vi "Validate Name Is Unique.vi"(8 "error in (no error)":errorcluster, 10 "Name in":string, 11 "Parent Ref in":T1=18446744073709551615 format="%.0x") -> (0 "error out":errorcluster, 1 "Unique?":bool, 2 "Name out":string, 3 "Parent Ref out":T1=18446744073709551615 format="%.0x")   [LabVIEW 2018, in "Instrument Addon Scripting API.lvlib"]
uses:
  Instrument Addon Scripting API.lvlib
  <vilib>/NI Veristand/Custom Device API/Custom Device Item Ref.ctl
  <vilib>/NI Veristand/Custom Device Tools/Custom Device Utility Library/Custom Device Utility Library.lvlib
  <vilib>/NI Veristand/Custom Device API/Custom Device API.lvlib
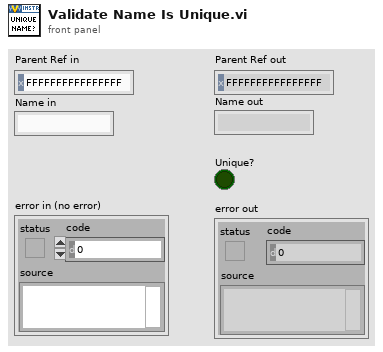
[diagram p1: front panel]
types:
  T1 = typedef "Custom Device API.lvlib/Custom Device Item Ref.ctl" = u64
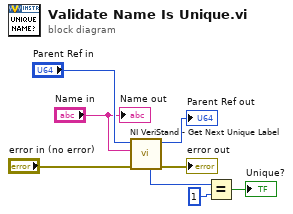
[diagram p0: block diagram]
diagram:
  n1 = call <vilib>:"NI VeriStand - Get Next Unique Label.vi"("error in (no error)"="error in (no error)", "Label"="Name in", "Parent Ref in"="Parent Ref in") -> ("error out"=→"error out":errorcluster, "Parent Ref dup"=→"Parent Ref out":T1, "Next value"=w3:i32)  [unwired: 5 in, 1 out]
  n2 = Equal?(x=w3, y=1) -> (x = y?=→"Unique?":bool)
  "Name out" <- "Name in"
